vi "elementAtGoalieArea+.vi"(7 "Elemento pos.":dbl[](array[numeric]), 8 "error in (no error)":errorcluster, 10 "Game":refnum<class "Game.lvclass">, 11 "Utilities in":refnum<class "Utilities.lvclass">) -> (0 "error out":errorcluster, 2 "Elemento at goalkeeper area + ?":bool, 3 "Utilities out":refnum<class "Utilities.lvclass">)   [LabVIEW 2023, in "Utilities.lvclass"]
uses:
  Utilities.lvclass
  Game_class/Game.lvclass
  Game_class/Game.lvclass/Game.ctl
  Parameters_class/Parameters.lvclass/Parameters.ctl
  Parameters_class/Read Area.vi
  Game_class/Read FieldRef.vi
  Game_class/Read Parameters.lvclass.vi
  Field_class/Field.lvclass
  Parameters_class/Parameters.lvclass
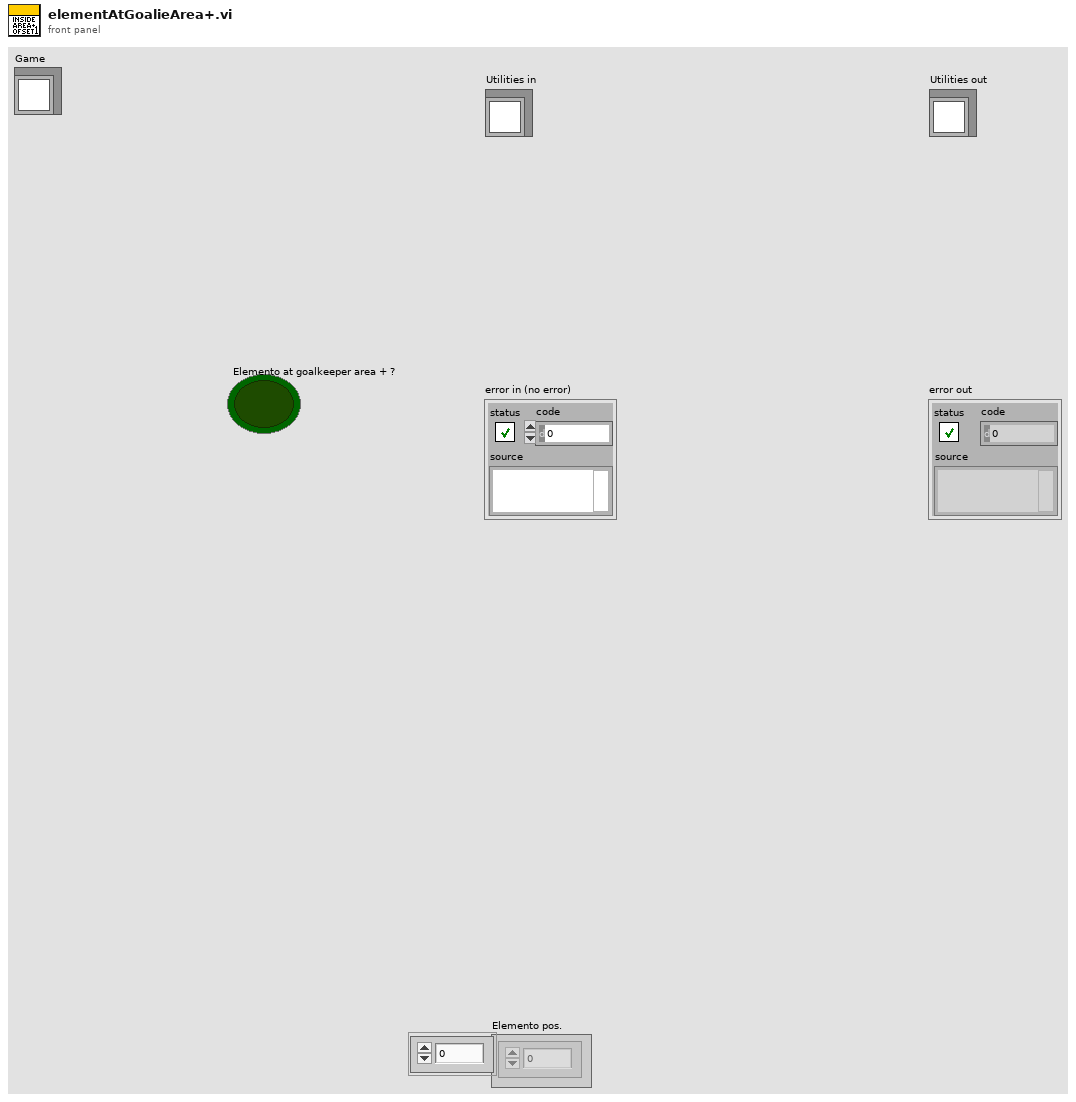
[diagram p1: front panel]
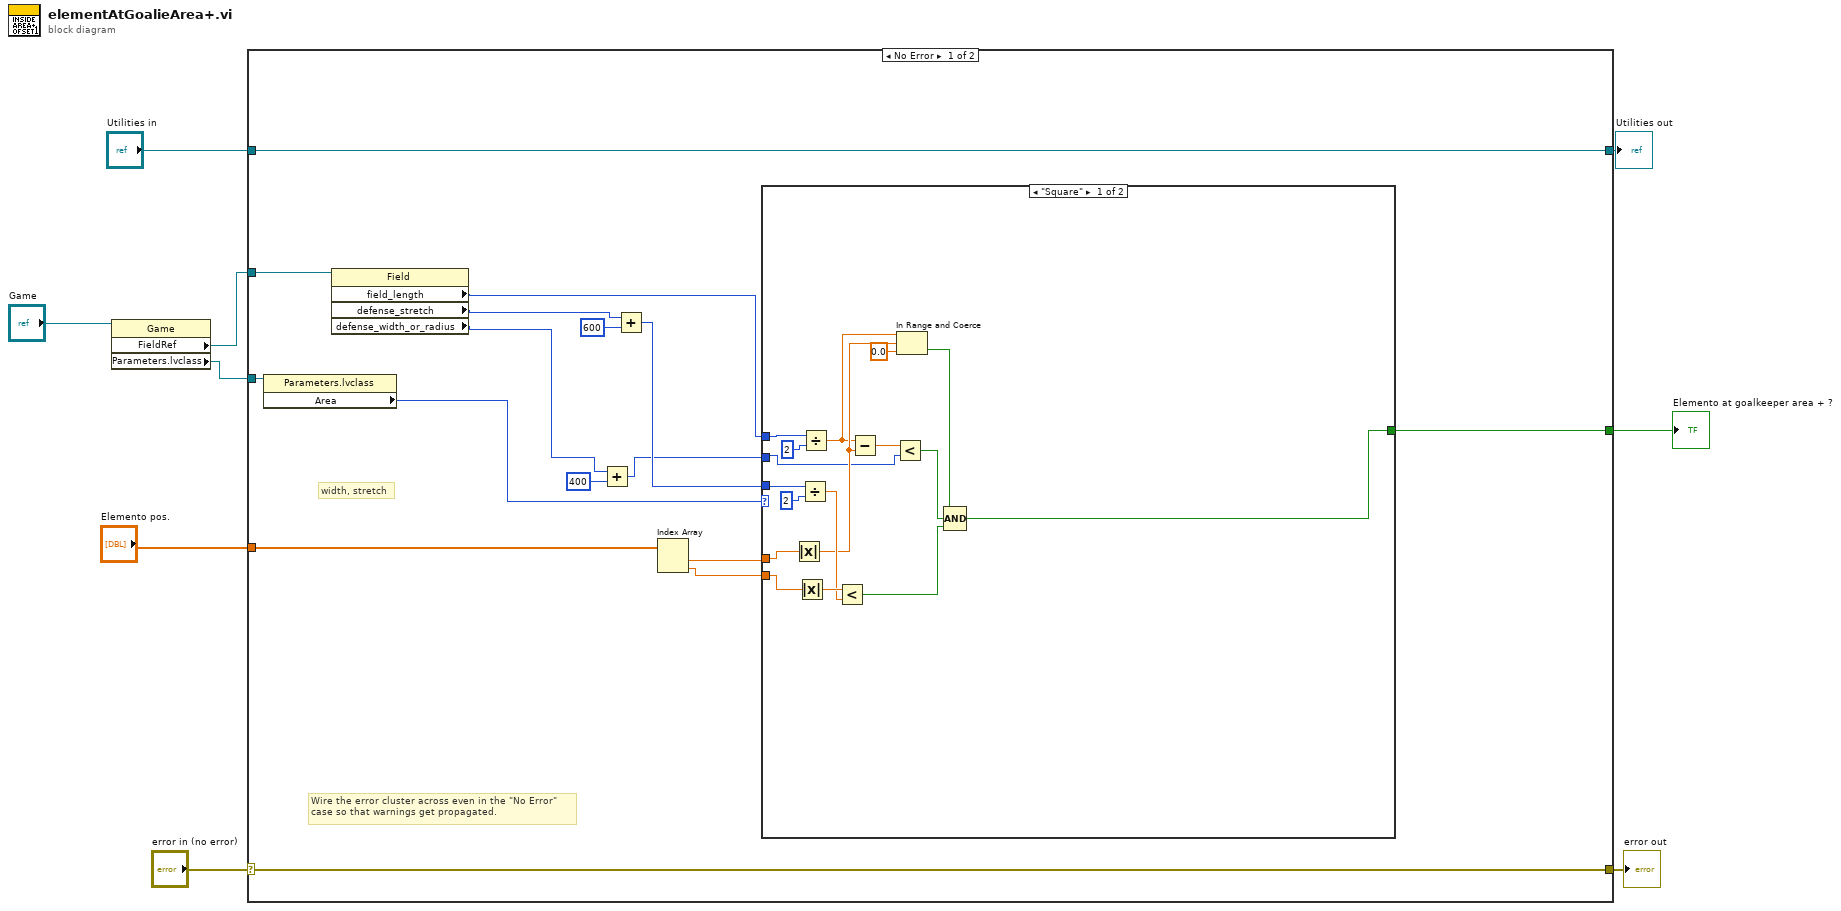
[diagram p0: block diagram]
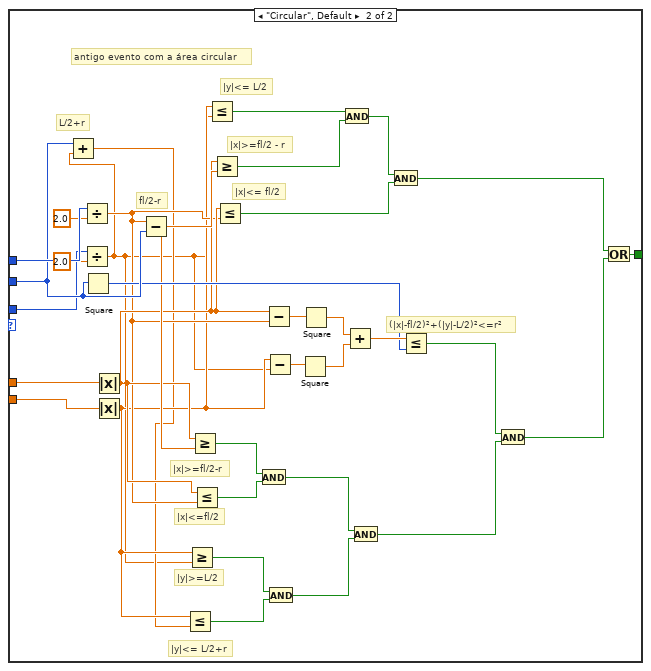
[diagram p2: hidden frame]
diagram:
  n1 = property class="Game"(reference="Game") -> ("FieldRef"=w3:refnum<class "Field.lvclass">, "Parameters.lvclass"=w2:refnum<class "Parameters.lvclass">)  [unwired: 1 in, 2 out]
  n2 = case shown="No Error" "error in (no error)" {
    selector: "error in (no error)" -> [w24 w78]
    tunnel: [w24 w78] -> w8
    tunnel: [w25 w77] -> w6
    tunnel: "Utilities in" -> [w25 w77]
    tunnel: w3 -> [w17 _]
    tunnel: "Elemento pos." -> [w16 _]
    tunnel: [w15 _] -> w4
    tunnel: w2 -> [w14 _]
    frame No Error {
      # "width, stretch"
      # "Wire the error cluster across even in the \"No Error\"\ncase so that warnings get propagated."
      n3 = property class="Parameters.lvclass"(reference=w14) -> ("Area"=w13:enum16{"Circular", "Square"})  [unwired: 1 in, 2 out]
      n4 = property class="Field"(reference=w17) -> ("field_length"=w19:i32, "defense_stretch"=w18:i32, "defense_width_or_radius"=w11:i32)  [unwired: 1 in, 2 out]
      n5 = Add(x=w11, y=400) -> (x+y=w10:i32)
      n6 = Add(x=w18, y=u32 600) -> (x+y=w22:u32)
      n7 = Index Array(array=w16) -> (element #1=w20:dbl, element #2=w21:dbl)  [unwired: 2 in]
      n8 = case shown="\"Square\"" w13 {
        tunnel: w21 -> [w30 w76]
        tunnel: w20 -> [w31 w75]
        tunnel: w19 -> [w28 w74]
        tunnel: [w26 w73] -> w15
        tunnel: w10 -> [w27 w72]
        tunnel: w22 -> [w29 w71]
        frame "Square" {
          n9 = Absolute Value(x=w31) -> (abs(x)=w35:dbl)
          n10 = Absolute Value(x=w30) -> (abs(x)=w41:dbl)
          n11 = Divide(x=w29, y=u32 2) -> (x/y=w38:dbl)
          n12 = Divide(x=w28, y=u32 2) -> (x/y=w33:dbl)
          n13 = Less?(x=w41, y=w38) -> (x < y?=w36:bool)
          n14 = Subtract(x=w33, y=w35) -> (x-y=w40:dbl)
          n15 = Less?(x=w40, y=w27) -> (x < y?=w37:bool)
          n16 = In Range and Coerce(upper limit=w33, x=w35, lower limit=0.0) -> (In Range?=w32:bool)  [unwired: 1 out]
          n17 = Compound Arithmetic op=AND(w32, w37, w36) -> (w26:bool)
        }
        frame "Circular", Default {
          # "antigo evento com a área circular"
          # "|y|<= L/2+r"
          # "L/2+r"
          # "|y|>=L/2"
          # "|x|<=fl/2"
          # "|x|>=fl/2-r"
          # "fl/2-r"
          # "(|x|-fl/2)²+(|y|-L/2)²<=r²"
          # "|x|<= fl/2"
          # "|x|>=fl/2 - r"
          # "|y|<= L/2"
          n18 = Divide(x=w74, y=2.0) -> (x/y=w54:dbl)
          n19 = Divide(x=w71, y=2.0) -> (x/y=w43:dbl)
          n20 = Add(x=w72, y=w43) -> (x+y=w52:dbl)
          n21 = Square(x=w72) -> (x^2=w59:i32)
          n22 = Absolute Value(x=w75) -> (abs(x)=w57:dbl)
          n23 = Absolute Value(x=w76) -> (abs(x)=w53:dbl)
          n24 = Subtract(x=w54, y=w72) -> (x-y=w58:dbl)
          n25 = Less Or Equal?(x=w53, y=w52) -> (x <= y?=w50:bool)
          n26 = Greater Or Equal?(x=w53, y=w43) -> (x >= y?=w51:bool)
          n27 = Greater Or Equal?(x=w57, y=w58) -> (x >= y?=w56:bool)
          n28 = Less Or Equal?(x=w57, y=w54) -> (x <= y?=w55:bool)
          n29 = Less Or Equal?(x=w53, y=w43) -> (x <= y?=w68:bool)
          n30 = Greater Or Equal?(x=w57, y=w58) -> (x >= y?=w67:bool)
          n31 = Less Or Equal?(x=w57, y=w54) -> (x <= y?=w65:bool)
          n32 = And(x=w56, y=w55) -> (x .and. y?=w49:bool)
          n33 = Subtract(x=w57, y=w54) -> (x-y=w64:dbl)
          n34 = Subtract(x=w53, y=w43) -> (x-y=w63:dbl)
          n35 = And(x=w51, y=w50) -> (x .and. y?=w48:bool)
          n36 = Square(x=w63) -> (x^2=w61:dbl)
          n37 = Square(x=w64) -> (x^2=w62:dbl)
          n38 = And(x=w68, y=w67) -> (x .and. y?=w66:bool)
          n39 = Add(x=w62, y=w61) -> (x+y=w60:dbl)
          n40 = And(x=w49, y=w48) -> (x .and. y?=w46:bool)
          n41 = And(x=w66, y=w65) -> (x .and. y?=w45:bool)
          n42 = Less Or Equal?(x=w60, y=w59) -> (x <= y?=w47:bool)
          n43 = And(x=w47, y=w46) -> (x .and. y?=w44:bool)
          n44 = Or(x=w45, y=w44) -> (x .or. y?=w73:bool)
        }
      }
    }
    frame Error {
    }
  }
  "error out" <- w8
  "Utilities out" <- w6
  "Elemento at goalkeeper area + ?" <- w4
